vi "lab2labviewq2.vi"() -> ()   [LabVIEW 2025]
uses:
  <vilib>/Analysis/2dsp.llb/Real FFT.vi
  <vilib>/Analysis/3filter.llb/Butterworth Filter (DBL).vi
  <vilib>/measure/NI_MABase.lvlib
  <vilib>/Analysis/NI_AALPro.lvlib
  <vilib>/Analysis/NI_AALBase.lvlib
panel:
  in  "Numeric 7":dbl
  in  "Numeric 6":dbl
  in  "Numeric 5":dbl
  in  "Numeric 4":dbl
  out "Waveform Graph 3":dbl[](graph)
  out "Waveform Graph 2":dbl[](graph)
  in  "Numeric 3":dbl
  in  "Numeric 2":dbl
  in  "Numeric":dbl
  out "Waveform Graph":waveform(dbl)(graph)
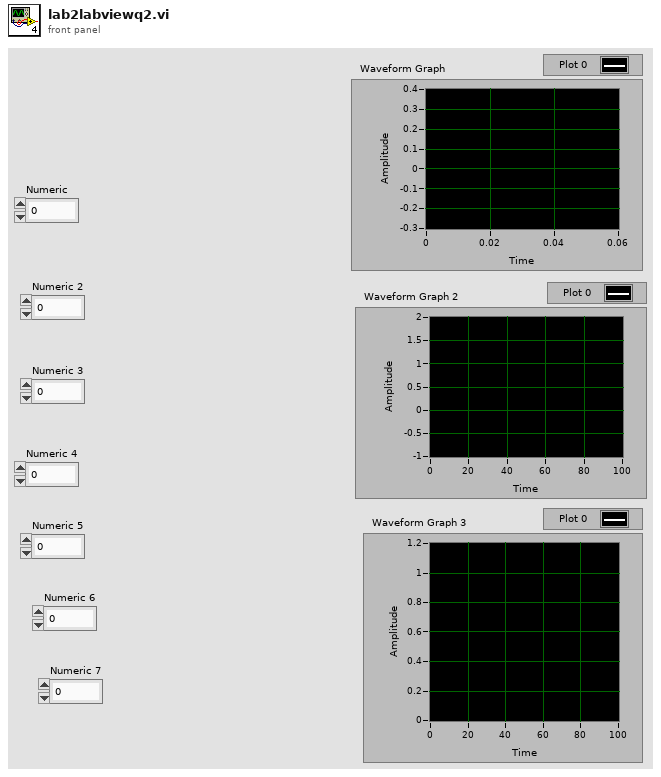
[diagram p1: front panel]
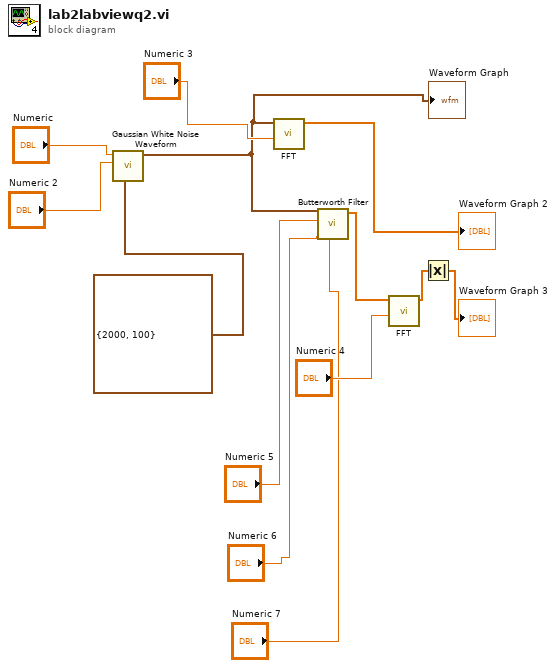
[diagram p0: block diagram]
diagram:
  n1 = call <vilib>:"Gaussian White Noise Waveform.vi"("sampling info"=cluster{i32, i32} {2000, 100}, "seed"="Numeric 2", "standard deviation"="Numeric") -> ("signal out"=w6:waveform(dbl))  [unwired: 7 in, 1 out]
  "Waveform Graph" <- w6
  n2 = call-poly <vilib>:"FFT.vi"("FFT size"="Numeric 3", "X"=w6) -> ("FFT {X}"=→"Waveform Graph 2":cdb[])  [unwired: 8 in, 1 out]
  n3 = call-poly <vilib>:"Butterworth Filter.vi"("order"="Numeric 7", "low cutoff freq: fl"="Numeric 6", "sampling freq: fs"="Numeric 5", "X"=w6) -> ("Filtered X"=w12:dbl[])  [unwired: 4 in, 1 out]
  n4 = call-poly <vilib>:"FFT.vi"("FFT size"="Numeric 4", "X"=w12) -> ("FFT {X}"=w2:cdb[])  [unwired: 8 in, 1 out]
  n5 = Absolute Value(x=w2) -> (abs(x)=→"Waveform Graph 3":dbl[])
